vi "Check Status No Objects - Spectrometer ActiveX.vi"(8 "error in (no error)":errorcluster, 11 "Spectrometer iHR320 in 2":T1={"Wavelength"=0.0, "Entrance slit width"=0.0, "Exit slit width"=0.0, "Init"={"Initialized?"=FALSE, "Emulating?"=FALSE}, "Grating"={"Groove Density"=0.0, "Blaze Wavelength"="", "Turrent Position"=0}, "RefNum"=refnum, "Unique ID"="", "FW RefNum"=refnum, "FW Unique ID"="", "Filter Index"=1} {"Grating"."Turrent Position" items=["Grating 1"=1, "Grating 2"=2]; "Filter Index" items=["Filter 1"=1, "Empty"=2, "Empty"=3, "Empty"=4, "Filter 2"=5, "Filter 3"=6]}) -> (0 "error out":errorcluster, 1 "Status":string, 2 "Ready?":bool, 3 "Spectrometer iHR320 out":T1={"Wavelength"=0.0, "Entrance slit width"=0.0, "Exit slit width"=0.0, "Init"={"Initialized?"=FALSE, "Emulating?"=FALSE}, "Grating"={"Groove Density"=0.0, "Blaze Wavelength"="", "Turrent Position"=0}, "RefNum"=refnum, "Unique ID"="", "FW RefNum"=refnum, "FW Unique ID"="", "Filter Index"=1} {"Grating"."Turrent Position" items=["Grating 1"=1, "Grating 2"=2]; "Filter Index" items=["Filter 1"=1, "Empty"=2, "Empty"=3, "Empty"=4, "Filter 2"=5, "Filter 3"=6]})   [LabVIEW 2012]
doc: "(Dynamic) Check if the instrument is powered on and update its member fields with the instrument's current status. Optionally return a text status message."
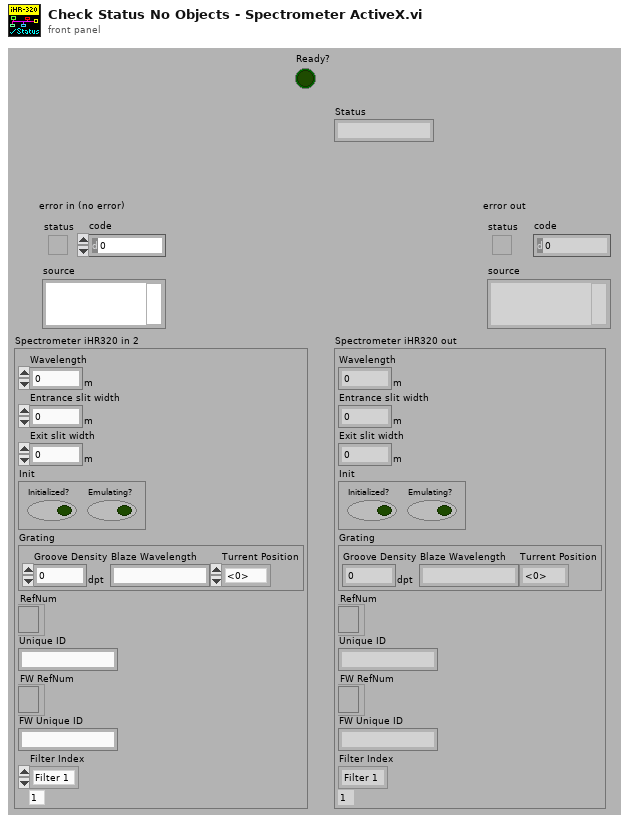
[diagram p1: front panel]
types:
  T1 = cluster{"Wavelength":dbl[unit], "Entrance slit width":dbl[unit], "Exit slit width":dbl[unit], "Init":cluster{"Initialized?":bool, "Emulating?":bool}, "Grating":cluster{"Groove Density":dbl[unit], "Blaze Wavelength":string, "Turrent Position":u16}, "RefNum":refnum<k7>, "Unique ID":string, "FW RefNum":refnum<k7>, "FW Unique ID":string, "Filter Index":i32}
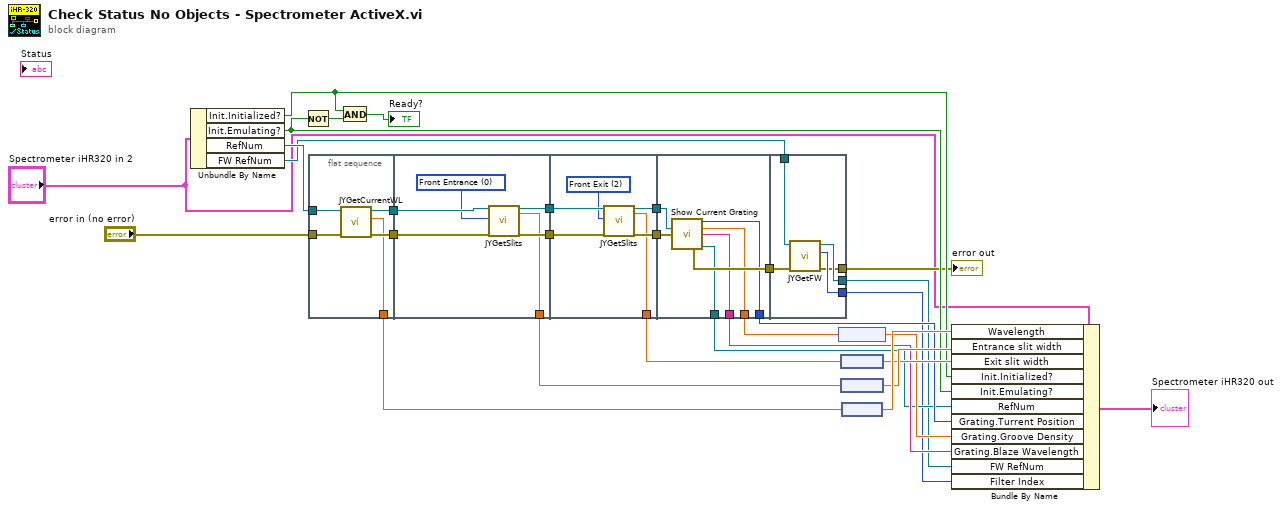
[diagram p0: block diagram]
diagram:
  n1 = Unbundle By Name("Spectrometer iHR320 in 2") -> ("Init.Initialized?"=w23:bool, "Init.Emulating?"=w24:bool, "RefNum"=w22:refnum<k7>, "FW RefNum"=w14:refnum<k7>)
  n2 = Not(x=w24) -> (.not. x?=w25:bool)
  n3 = flat-sequence {
    tunnel: w22 -> [w35]
    tunnel: "error in (no error)" -> [w34]
    tunnel: [w33] -> w21
    tunnel: [w32] -> w18
    tunnel: [w31] -> w13
    tunnel: w21 -> [w41]
    tunnel: [w40] -> w20
    tunnel: w18 -> [w39]
    tunnel: [w38] -> w17
    tunnel: [w37] -> w12
    tunnel: w20 -> [w47]
    tunnel: [w46] -> w19
    tunnel: w17 -> [w45]
    tunnel: [w44] -> w16
    tunnel: [w43] -> w11
    tunnel: w19 -> [w54]
    tunnel: w16 -> [w53]
    tunnel: [w52] -> w15
    tunnel: [w51] -> w10
    tunnel: [w50] -> w9
    tunnel: [w49] -> w8
    tunnel: [w48] -> w7
    tunnel: w15 -> [w59]
    tunnel: w14 -> [w58]
    tunnel: [w57] -> w6
    tunnel: [w56] -> w5
    tunnel: [w55] -> w4
    frame #0 {
      n4 = call "JYGetCurrentWL.vi"("error in (no error)"=w34, "JYMONOLib.IJYMonoReqd In"=w35) -> ("error out"=w32:errorcluster, "Current WL"=w31:dbl, "JYMONOLib.IJYMonoReqd Out"=w33:refnum<k7>)  [unwired: 6 in, 1 out]
    }
    frame #1 {
      w36 = u16 0 items=["Front Entrance", "Side Entrance", "Front Exit", "Side Exit", "First Intermediate", "Second Intermediate"] ("Slit")
      n5 = call "JYGetSlits.vi"("MonoRefNum IN"=w41, "Slit"=w36, "error in (no error)"=w39) -> ("MonoRefNum Out"=w40:refnum<k7>, "Slit Width"=w37:dbl, "error out"=w38:errorcluster)  [unwired: 13 in, 1 out]
    }
    frame #2 {
      w42 = u16 2 items=["Front Entrance", "Side Entrance", "Front Exit", "Side Exit", "First Intermediate", "Second Intermediate"] ("Slit")
      n6 = call "JYGetSlits.vi"("MonoRefNum IN"=w47, "Slit"=w42, "error in (no error)"=w45) -> ("MonoRefNum Out"=w46:refnum<k7>, "Slit Width"=w43:dbl, "error out"=w44:errorcluster)  [unwired: 13 in, 1 out]
    }
    frame #3 {
      n7 = call "Show Current Grating.vi"("JYMONOLib.IJYMonoReqd  in"=w54, "error in (no error)"=w53) -> ("Grating Index"=w49:i32, "Current Grating"=w51:dbl, "Current Blaze"=w50:string, "error out"=w52:errorcluster, "JYMONOLib.IJYMonoReqd Out"=w48:refnum<k7>)  [unwired: 5 in, 4 out]
    }
    frame #4 {
      n8 = call "JYGetFW.vi"("error in (no error)"=w59, "FW RefNum In"=w58) -> ("error out"=w55:errorcluster, "Filter Index"=w56:i32, "FW RefNum Out"=w57:refnum<k7>)  [unwired: 7 in]
    }
  }
  n9 = And(x=w23, y=w25) -> (x .and. y?=→"Ready?":bool)
  n10 = node(w10) -> (w27:dbl[unit])
  n11 = node(w11) -> (w28:dbl[unit])
  n12 = node(w12) -> (w29:dbl[unit])
  n13 = node(w13) -> (w30:dbl[unit])
  n14 = Bundle By Name(cluster="Spectrometer iHR320 in 2", "Wavelength"=w30, "Entrance slit width"=w29, "Exit slit width"=w28, "Init.Initialized?"=w23, "Init.Emulating?"=w24, "RefNum"=w7, "Grating.Turrent Position"=w8, "Grating.Groove Density"=w27, "Grating.Blaze Wavelength"=w9, "FW RefNum"=w6, "Filter Index"=w5) -> (→"Spectrometer iHR320 out":T1)
  "error out" <- w4
